vi "Search_Dust_Types.vi"() -> ()   [LabVIEW 2013]
doc: "Searches the dust_type table for a user-selected dust name. For use in the Dust Lab. All results can be ordered by id_dust_type, dust name, density, source mass, bottle mass, or dust mass."
uses:
  <userlib>/Accelerator/User Interface/Controls/Dust_list.ctl
  <vilib>/Utility/miscctls.llb/LVPointTypeDef.ctl
panel:
  out "Descending":string
  out "Ascending":string
  out "dust_weight text":string
  out "bottle_weight text":string
  out "source_weight text":string
  out "dust_density text":string
  out "dust_name text":string
  out "id_dust_type text":string
  in  "Exit":bool
  out "error out":errorcluster
  in  "error in (no error)":errorcluster
  in  "dust_weight":bool
  in  "bottle_weight":bool
  in  "source_weight":bool
  in  "dust_density":bool
  in  "dust_name":bool
  in  "id_dust_type":bool
  out "Array":T1[](array[typedef])
  # "Size"
  # "Comments"
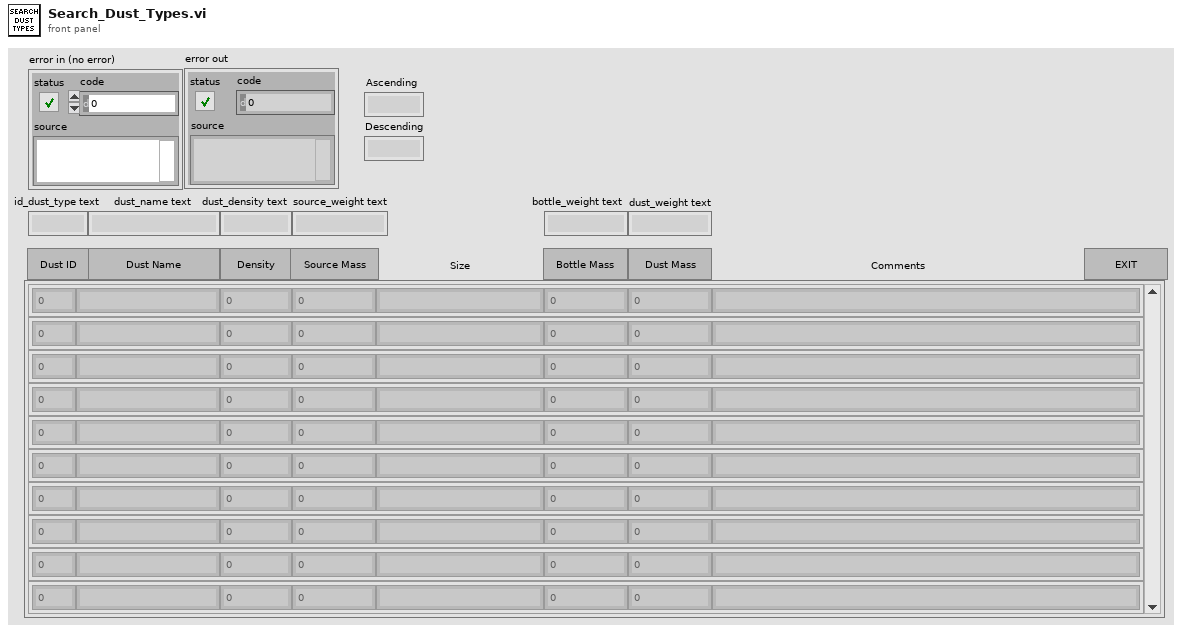
[diagram p1: front panel]
types:
  T1 = typedef "Dust_list.ctl" = cluster{"id_dust_type":i32, "dust_name":string, "dust_type":i32, "batch_no":i32, "dust_density":dbl, "source_weight":dbl, "size":string, "bottle_weight":dbl, "dust_mass":dbl, "comments":string}
  T2 = typedef "LVPointTypeDef.ctl" = cluster{"Horizontal":i16, "Vertical":i16}
  T3 = enum16{"dust_name", "dust_density", "source_weight", "bottle_weight", "dust_weight"}
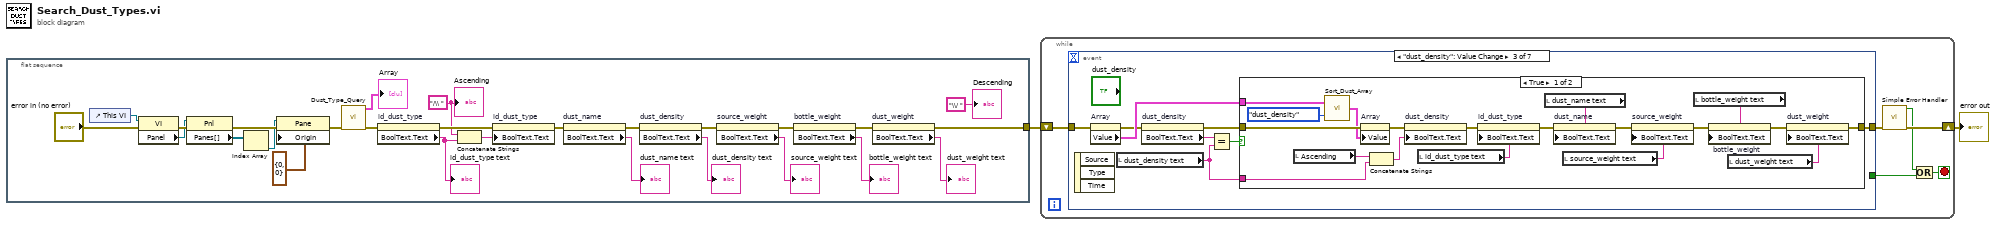
[diagram p0: block diagram]
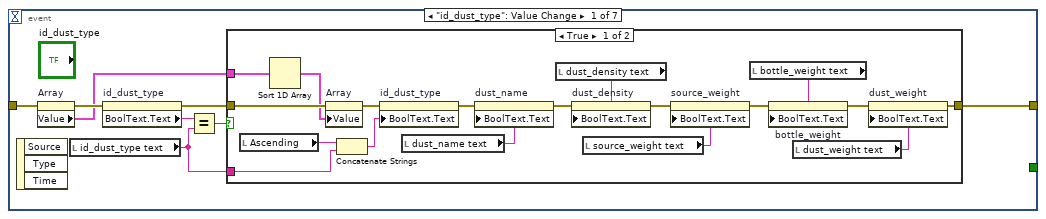
[diagram p2: hidden frame]
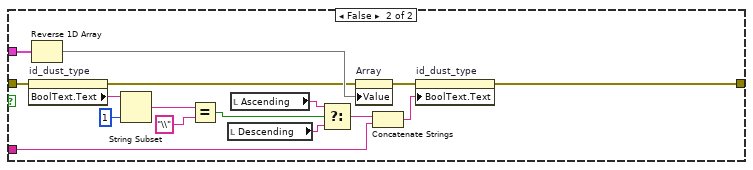
[diagram p3: hidden frame]
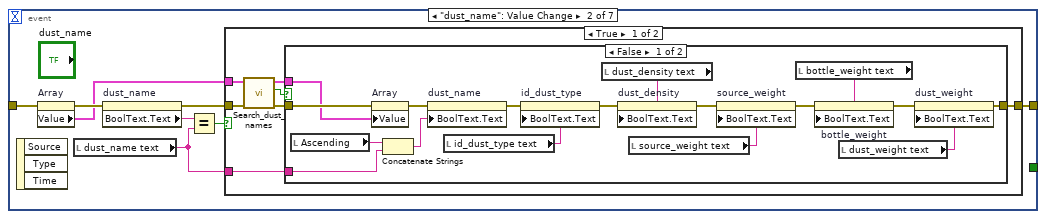
[diagram p4: hidden frame]
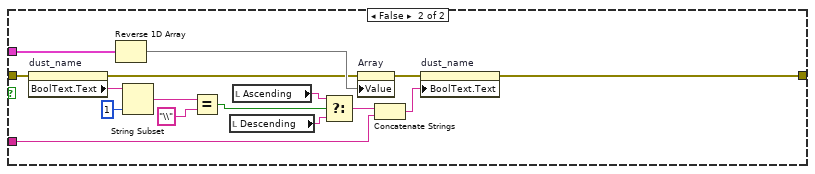
[diagram p6: hidden frame]
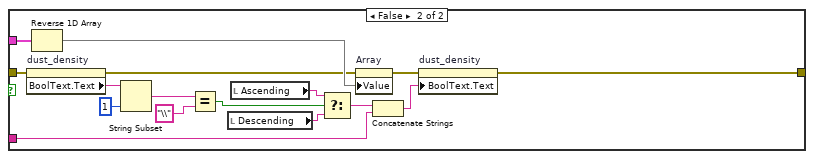
[diagram p7: hidden frame]
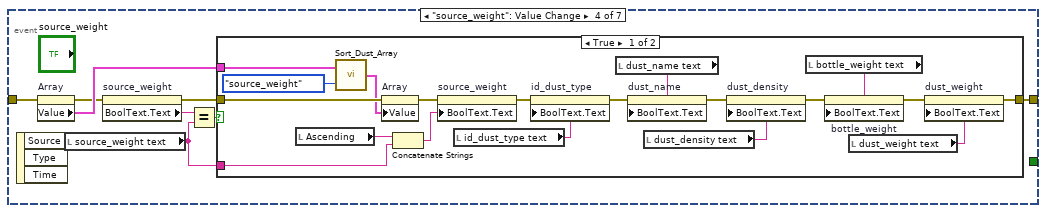
[diagram p8: hidden frame]
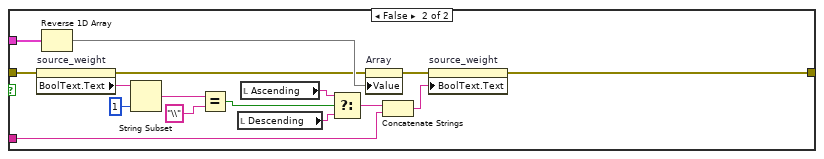
[diagram p9: hidden frame]
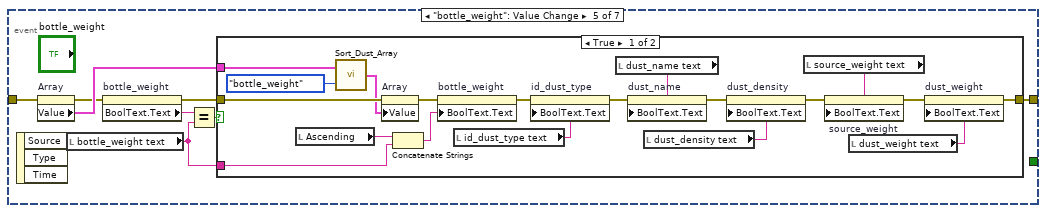
[diagram p10: hidden frame]
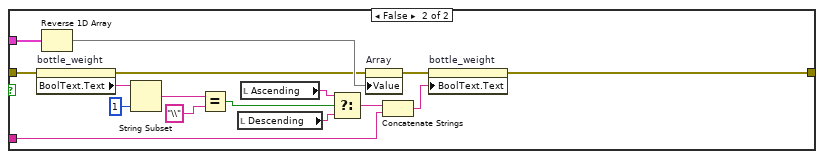
[diagram p11: hidden frame]
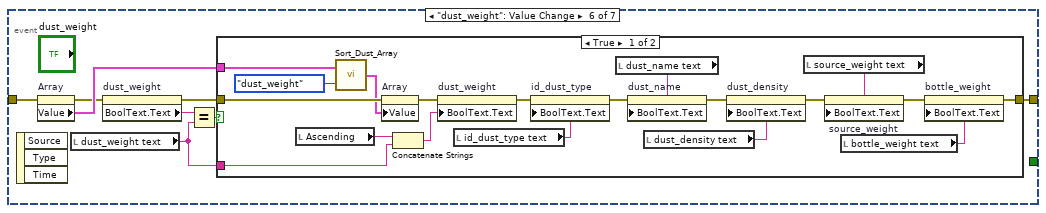
[diagram p12: hidden frame]
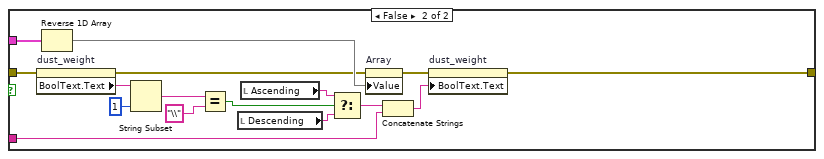
[diagram p13: hidden frame]
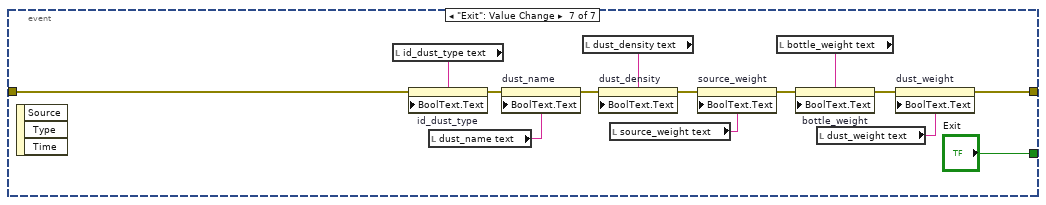
[diagram p14: hidden frame]
diagram:
  n1 = flat-sequence {
    tunnel: [w20] -> w1
    frame #0 {
      w3 = "/\\ " ("Ascending")
      n2 = control-ref of="This VI"() -> (w15:refnum<vi>)
      n3 = property class="VI"(reference=w15, error in="error in (no error)") -> (error out=w14:errorcluster, "Panel"=w13:refnum<vi>)  [unwired: 1 out]
      n4 = property class="Pnl"(reference=w13, error in=w14) -> (error out=w12:errorcluster, "Panes[]"=w11:refnum<vi>[])  [unwired: 1 out]
      n5 = Index Array(array=w11) -> (element=w10:refnum<vi>)  [unwired: 1 in]
      n6 = property class="Pane"(reference=w10, error in=w12, "Origin"=T2 {"Horizontal"=0, "Vertical"=0}) -> (error out=w8:errorcluster)  [unwired: 1 out]
      n7 = call <userlib>:"Dust_Type_Query.vi"("error in (no error)"=w8) -> ("error out"=w18:errorcluster, "Dust Type Array"=→"Array":T1[])  [unwired: 9 in]
      n8 = property on="id_dust_type" class="Bool"(error in=w18) -> (error out=w6:errorcluster, "BoolText.Text"=w4:string)  [unwired: 1 in, 1 out]
      "id_dust_type text" <- w4
      n9 = Concatenate Strings(w3, w4) -> (w5:string)
      n10 = property on="id_dust_type" class="Bool"(error in=w6, "BoolText.Text"=w5) -> (error out=w7:errorcluster)  [unwired: 1 in, 1 out]
      n11 = property on="dust_name" class="Bool"(error in=w7) -> (error out=w29:errorcluster, "BoolText.Text"=→"dust_name text":string)  [unwired: 1 in, 1 out]
      n12 = property on="dust_density" class="Bool"(error in=w29) -> (error out=w26:errorcluster, "BoolText.Text"=→"dust_density text":string)  [unwired: 1 in, 1 out]
      n13 = property on="source_weight" class="Bool"(error in=w26) -> (error out=w24:errorcluster, "BoolText.Text"=→"source_weight text":string)  [unwired: 1 in, 1 out]
      n14 = property on="bottle_weight" class="Bool"(error in=w24) -> (error out=w22:errorcluster, "BoolText.Text"=→"bottle_weight text":string)  [unwired: 1 in, 1 out]
      n15 = property on="dust_weight" class="Bool"(error in=w22) -> (error out=w20:errorcluster, "BoolText.Text"=→"dust_weight text":string)  [unwired: 1 in, 1 out]
      "Ascending" <- w3
      "Descending" <- "\\/ " ("Descending")
    }
  }
  n16 = while {
    shift-right: [w32] -> w2
    shift-left: w1 -> [w35]
    stop <- w31 stop-if-true
    n17 = event shown="[2] \"dust_density\": Value Change" {
      selector: _ -> [_ _ _ _ _ _ _]
      dyn-events: _ -> [_ _ _ _ _ _ _]
      timeout: _ -> [_ _ _ _ _ _ _]
      tunnel: w35 -> [w43 w85 w134 w177 w220 w263 w306]
      tunnel: [w42 w84 w133 w176 w219 w262 w305] -> w34
      tunnel: [_ _ _ _ _ _ "Exit"] -> w33
      event "id_dust_type": Value Change {
        n18 = event-data() -> ()  [unwired: 1 in, 3 out]
        n19 = property on="Array" class="Arr (strict)"(error in=w43) -> (error out=w37:errorcluster, "Value"=w36:T1[])  [unwired: 1 in, 1 out]
        n20 = local read "id_dust_type text"() -> (w40:string)
        n21 = property on="id_dust_type" class="Bool"(error in=w37) -> (error out=w38:errorcluster, "BoolText.Text"=w41:string)  [unwired: 1 in, 1 out]
        n22 = Equal?(x=w41, y=w40) -> (x = y?=w39:bool)
        n23 = case shown="True" w39 {
          tunnel: [w48 w76] -> w42
          tunnel: w40 -> [w59 w75]
          tunnel: w38 -> [w47 w64]
          tunnel: w36 -> [w45 w74]
          frame True {
            n24 = local read "Ascending"() -> (w60:string)
            n25 = Sort 1D Array(array=w45) -> (sorted array=w44:T1[])
            n26 = property on="Array" class="Arr (strict)"(error in=w47, "Value"=w44) -> (error out=w46:errorcluster)  [unwired: 1 in, 1 out]
            n27 = Concatenate Strings(w60, w59) -> (w61:string)
            n28 = property on="id_dust_type" class="Bool"(error in=w46, "BoolText.Text"=w61) -> (error out=w49:errorcluster)  [unwired: 1 in, 1 out]
            n29 = local read "dust_name text"() -> (w53:string)
            n30 = property on="dust_name" class="Bool"(error in=w49, "BoolText.Text"=w53) -> (error out=w54:errorcluster)  [unwired: 1 in, 1 out]
            n31 = local read "dust_density text"() -> (w52:string)
            n32 = property on="dust_density" class="Bool"(error in=w54, "BoolText.Text"=w52) -> (error out=w55:errorcluster)  [unwired: 1 in, 1 out]
            n33 = local read "source_weight text"() -> (w51:string)
            n34 = property on="source_weight" class="Bool"(error in=w55, "BoolText.Text"=w51) -> (error out=w56:errorcluster)  [unwired: 1 in, 1 out]
            n35 = local read "bottle_weight text"() -> (w50:string)
            n36 = property on="bottle_weight" class="Bool"(error in=w56, "BoolText.Text"=w50) -> (error out=w57:errorcluster)  [unwired: 1 in, 1 out]
            n37 = local read "dust_weight text"() -> (w58:string)
            n38 = property on="dust_weight" class="Bool"(error in=w57, "BoolText.Text"=w58) -> (error out=w48:errorcluster)  [unwired: 1 in, 1 out]
          }
          frame False {
            n39 = property on="id_dust_type" class="Bool"(error in=w64) -> (error out=w63:errorcluster, "BoolText.Text"=w70:string)  [unwired: 1 in, 1 out]
            n40 = Reverse 1D Array(array=w74) -> (reversed array=w73:T1[])
            n41 = String Subset(string=w70, length (rest)=1 ("length (rest)")) -> (substring=w67:string)  [unwired: 1 in]
            n42 = Equal?(x=w67, y="\\") -> (x = y?=w65:bool)
            n43 = local read "Descending"() -> (w72:string)
            n44 = local read "Ascending"() -> (w68:string)
            n45 = Select(t=w68, s=w65, f=w72) -> (s? t:f=w71:string)
            n46 = property on="Array" class="Arr (strict)"(error in=w63, "Value"=w73) -> (error out=w62:errorcluster)  [unwired: 1 in, 1 out]
            n47 = Concatenate Strings(w71, w75) -> (w77:string)
            n48 = property on="id_dust_type" class="Bool"(error in=w62, "BoolText.Text"=w77) -> (error out=w76:errorcluster)  [unwired: 1 in, 1 out]
          }
        }
      }
      event "dust_name": Value Change {
        n49 = event-data() -> ()  [unwired: 1 in, 3 out]
        n50 = property on="Array" class="Arr (strict)"(error in=w85) -> (error out=w81:errorcluster, "Value"=w79:T1[])  [unwired: 1 in, 1 out]
        n51 = local read "dust_name text"() -> (w83:string)
        n52 = property on="dust_name" class="Bool"(error in=w81) -> (error out=w78:errorcluster, "BoolText.Text"=w80:string)  [unwired: 1 in, 1 out]
        n53 = Equal?(x=w80, y=w83) -> (x = y?=w82:bool)
        n54 = case shown="True" w82 {
          tunnel: [w91 w112] -> w84
          tunnel: w83 -> [w92 w126]
          tunnel: w78 -> [w90 w116]
          tunnel: w79 -> [w88 w125]
          frame True {
            n55 = call <userlib>:"Search_dust_names.vi"("error in (no error)"=w90, "Dust array in"=w88) -> ("error out"=w89:errorcluster, "Cancelled?"=w86:bool, "Dust array out"=w87:T1[])  [unwired: 7 in]
            n56 = case shown="False" w86 {
              tunnel: w92 -> [w108 _]
              tunnel: [w98 w110] -> w91
              tunnel: w89 -> [w94 w110]
              tunnel: w87 -> [w93 _]
              frame False {
                n57 = local read "Ascending"() -> (w109:string)
                n58 = property on="Array" class="Arr (strict)"(error in=w94, "Value"=w93) -> (error out=w96:errorcluster)  [unwired: 1 in, 1 out]
                n59 = Concatenate Strings(w109, w108) -> (w95:string)
                n60 = property on="dust_name" class="Bool"(error in=w96, "BoolText.Text"=w95) -> (error out=w97:errorcluster)  [unwired: 1 in, 1 out]
                n61 = local read "id_dust_type text"() -> (w102:string)
                n62 = property on="id_dust_type" class="Bool"(error in=w97, "BoolText.Text"=w102) -> (error out=w103:errorcluster)  [unwired: 1 in, 1 out]
                n63 = local read "dust_density text"() -> (w101:string)
                n64 = property on="dust_density" class="Bool"(error in=w103, "BoolText.Text"=w101) -> (error out=w104:errorcluster)  [unwired: 1 in, 1 out]
                n65 = local read "source_weight text"() -> (w100:string)
                n66 = property on="source_weight" class="Bool"(error in=w104, "BoolText.Text"=w100) -> (error out=w105:errorcluster)  [unwired: 1 in, 1 out]
                n67 = local read "bottle_weight text"() -> (w99:string)
                n68 = property on="bottle_weight" class="Bool"(error in=w105, "BoolText.Text"=w99) -> (error out=w106:errorcluster)  [unwired: 1 in, 1 out]
                n69 = local read "dust_weight text"() -> (w107:string)
                n70 = property on="dust_weight" class="Bool"(error in=w106, "BoolText.Text"=w107) -> (error out=w98:errorcluster)  [unwired: 1 in, 1 out]
              }
              frame True {
              }
            }
          }
          frame False {
            n71 = property on="dust_name" class="Bool"(error in=w116) -> (error out=w115:errorcluster, "BoolText.Text"=w114:string)  [unwired: 1 in, 1 out]
            n72 = Reverse 1D Array(array=w125) -> (reversed array=w124:T1[])
            n73 = String Subset(string=w114, length (rest)=1 ("length (rest)")) -> (substring=w119:string)  [unwired: 1 in]
            n74 = Equal?(x=w119, y="\\") -> (x = y?=w117:bool)
            n75 = local read "Descending"() -> (w123:string)
            n76 = local read "Ascending"() -> (w120:string)
            n77 = Select(t=w120, s=w117, f=w123) -> (s? t:f=w122:string)
            n78 = property on="Array" class="Arr (strict)"(error in=w115, "Value"=w124) -> (error out=w113:errorcluster)  [unwired: 1 in, 1 out]
            n79 = Concatenate Strings(w122, w126) -> (w111:string)
            n80 = property on="dust_name" class="Bool"(error in=w113, "BoolText.Text"=w111) -> (error out=w112:errorcluster)  [unwired: 1 in, 1 out]
          }
        }
      }
      event "dust_density": Value Change {
        n81 = event-data() -> ()  [unwired: 1 in, 3 out]
        n82 = property on="Array" class="Arr (strict)"(error in=w134) -> (error out=w129:errorcluster, "Value"=w130:T1[])  [unwired: 1 in, 1 out]
        n83 = local read "dust_density text"() -> (w132:string)
        n84 = property on="dust_density" class="Bool"(error in=w129) -> (error out=w127:errorcluster, "BoolText.Text"=w128:string)  [unwired: 1 in, 1 out]
        n85 = Equal?(x=w128, y=w132) -> (x = y?=w131:bool)
        n86 = case shown="True" w131 {
          tunnel: [w142 w155] -> w133
          tunnel: w132 -> [w152 w169]
          tunnel: w127 -> [w141 w159]
          tunnel: w130 -> [w140 w168]
          frame True {
            n87 = local read "Ascending"() -> (w153:string)
            n88 = call <userlib>:"Sort_Dust_Array.vi"("Order by..."=T3."dust_density", "Array In"=w140) -> ("Array out"=w139:T1[])
            n89 = property on="Array" class="Arr (strict)"(error in=w141, "Value"=w139) -> (error out=w137:errorcluster)  [unwired: 1 in, 1 out]
            n90 = Concatenate Strings(w153, w152) -> (w136:string)
            n91 = property on="dust_density" class="Bool"(error in=w137, "BoolText.Text"=w136) -> (error out=w138:errorcluster)  [unwired: 1 in, 1 out]
            n92 = local read "id_dust_type text"() -> (w146:string)
            n93 = property on="id_dust_type" class="Bool"(error in=w138, "BoolText.Text"=w146) -> (error out=w147:errorcluster)  [unwired: 1 in, 1 out]
            n94 = local read "dust_name text"() -> (w145:string)
            n95 = property on="dust_name" class="Bool"(error in=w147, "BoolText.Text"=w145) -> (error out=w148:errorcluster)  [unwired: 1 in, 1 out]
            n96 = local read "source_weight text"() -> (w144:string)
            n97 = property on="source_weight" class="Bool"(error in=w148, "BoolText.Text"=w144) -> (error out=w149:errorcluster)  [unwired: 1 in, 1 out]
            n98 = local read "bottle_weight text"() -> (w143:string)
            n99 = property on="bottle_weight" class="Bool"(error in=w149, "BoolText.Text"=w143) -> (error out=w150:errorcluster)  [unwired: 1 in, 1 out]
            n100 = local read "dust_weight text"() -> (w151:string)
            n101 = property on="dust_weight" class="Bool"(error in=w150, "BoolText.Text"=w151) -> (error out=w142:errorcluster)  [unwired: 1 in, 1 out]
          }
          frame False {
            n102 = property on="dust_density" class="Bool"(error in=w159) -> (error out=w158:errorcluster, "BoolText.Text"=w157:string)  [unwired: 1 in, 1 out]
            n103 = Reverse 1D Array(array=w168) -> (reversed array=w167:T1[])
            n104 = String Subset(string=w157, length (rest)=1 ("length (rest)")) -> (substring=w162:string)  [unwired: 1 in]
            n105 = Equal?(x=w162, y="\\") -> (x = y?=w160:bool)
            n106 = local read "Descending"() -> (w166:string)
            n107 = local read "Ascending"() -> (w163:string)
            n108 = Select(t=w163, s=w160, f=w166) -> (s? t:f=w165:string)
            n109 = property on="Array" class="Arr (strict)"(error in=w158, "Value"=w167) -> (error out=w156:errorcluster)  [unwired: 1 in, 1 out]
            n110 = Concatenate Strings(w165, w169) -> (w154:string)
            n111 = property on="dust_density" class="Bool"(error in=w156, "BoolText.Text"=w154) -> (error out=w155:errorcluster)  [unwired: 1 in, 1 out]
          }
        }
      }
      event "source_weight": Value Change {
        n112 = event-data() -> ()  [unwired: 1 in, 3 out]
        n113 = property on="Array" class="Arr (strict)"(error in=w177) -> (error out=w172:errorcluster, "Value"=w173:T1[])  [unwired: 1 in, 1 out]
        n114 = local read "source_weight text"() -> (w175:string)
        n115 = property on="source_weight" class="Bool"(error in=w172) -> (error out=w170:errorcluster, "BoolText.Text"=w171:string)  [unwired: 1 in, 1 out]
        n116 = Equal?(x=w171, y=w175) -> (x = y?=w174:bool)
        n117 = case shown="True" w174 {
          tunnel: [w185 w198] -> w176
          tunnel: w175 -> [w195 w212]
          tunnel: w170 -> [w184 w202]
          tunnel: w173 -> [w183 w211]
          frame True {
            n118 = local read "Ascending"() -> (w196:string)
            n119 = call <userlib>:"Sort_Dust_Array.vi"("Order by..."=T3."source_weight", "Array In"=w183) -> ("Array out"=w182:T1[])
            n120 = property on="Array" class="Arr (strict)"(error in=w184, "Value"=w182) -> (error out=w180:errorcluster)  [unwired: 1 in, 1 out]
            n121 = Concatenate Strings(w196, w195) -> (w179:string)
            n122 = property on="source_weight" class="Bool"(error in=w180, "BoolText.Text"=w179) -> (error out=w181:errorcluster)  [unwired: 1 in, 1 out]
            n123 = local read "id_dust_type text"() -> (w189:string)
            n124 = property on="id_dust_type" class="Bool"(error in=w181, "BoolText.Text"=w189) -> (error out=w190:errorcluster)  [unwired: 1 in, 1 out]
            n125 = local read "dust_name text"() -> (w188:string)
            n126 = property on="dust_name" class="Bool"(error in=w190, "BoolText.Text"=w188) -> (error out=w191:errorcluster)  [unwired: 1 in, 1 out]
            n127 = local read "dust_density text"() -> (w187:string)
            n128 = property on="dust_density" class="Bool"(error in=w191, "BoolText.Text"=w187) -> (error out=w192:errorcluster)  [unwired: 1 in, 1 out]
            n129 = local read "bottle_weight text"() -> (w186:string)
            n130 = property on="bottle_weight" class="Bool"(error in=w192, "BoolText.Text"=w186) -> (error out=w193:errorcluster)  [unwired: 1 in, 1 out]
            n131 = local read "dust_weight text"() -> (w194:string)
            n132 = property on="dust_weight" class="Bool"(error in=w193, "BoolText.Text"=w194) -> (error out=w185:errorcluster)  [unwired: 1 in, 1 out]
          }
          frame False {
            n133 = property on="source_weight" class="Bool"(error in=w202) -> (error out=w201:errorcluster, "BoolText.Text"=w200:string)  [unwired: 1 in, 1 out]
            n134 = Reverse 1D Array(array=w211) -> (reversed array=w210:T1[])
            n135 = String Subset(string=w200, length (rest)=1 ("length (rest)")) -> (substring=w205:string)  [unwired: 1 in]
            n136 = Equal?(x=w205, y="\\") -> (x = y?=w203:bool)
            n137 = local read "Descending"() -> (w209:string)
            n138 = local read "Ascending"() -> (w206:string)
            n139 = Select(t=w206, s=w203, f=w209) -> (s? t:f=w208:string)
            n140 = property on="Array" class="Arr (strict)"(error in=w201, "Value"=w210) -> (error out=w199:errorcluster)  [unwired: 1 in, 1 out]
            n141 = Concatenate Strings(w208, w212) -> (w197:string)
            n142 = property on="source_weight" class="Bool"(error in=w199, "BoolText.Text"=w197) -> (error out=w198:errorcluster)  [unwired: 1 in, 1 out]
          }
        }
      }
      event "bottle_weight": Value Change {
        n143 = event-data() -> ()  [unwired: 1 in, 3 out]
        n144 = property on="Array" class="Arr (strict)"(error in=w220) -> (error out=w215:errorcluster, "Value"=w216:T1[])  [unwired: 1 in, 1 out]
        n145 = local read "bottle_weight text"() -> (w218:string)
        n146 = property on="bottle_weight" class="Bool"(error in=w215) -> (error out=w213:errorcluster, "BoolText.Text"=w214:string)  [unwired: 1 in, 1 out]
        n147 = Equal?(x=w214, y=w218) -> (x = y?=w217:bool)
        n148 = case shown="True" w217 {
          tunnel: [w228 w241] -> w219
          tunnel: w218 -> [w238 w255]
          tunnel: w213 -> [w227 w245]
          tunnel: w216 -> [w226 w254]
          frame True {
            n149 = local read "Ascending"() -> (w239:string)
            n150 = call <userlib>:"Sort_Dust_Array.vi"("Order by..."=T3."bottle_weight", "Array In"=w226) -> ("Array out"=w225:T1[])
            n151 = property on="Array" class="Arr (strict)"(error in=w227, "Value"=w225) -> (error out=w223:errorcluster)  [unwired: 1 in, 1 out]
            n152 = Concatenate Strings(w239, w238) -> (w222:string)
            n153 = property on="bottle_weight" class="Bool"(error in=w223, "BoolText.Text"=w222) -> (error out=w224:errorcluster)  [unwired: 1 in, 1 out]
            n154 = local read "id_dust_type text"() -> (w232:string)
            n155 = property on="id_dust_type" class="Bool"(error in=w224, "BoolText.Text"=w232) -> (error out=w233:errorcluster)  [unwired: 1 in, 1 out]
            n156 = local read "dust_name text"() -> (w231:string)
            n157 = property on="dust_name" class="Bool"(error in=w233, "BoolText.Text"=w231) -> (error out=w234:errorcluster)  [unwired: 1 in, 1 out]
            n158 = local read "dust_density text"() -> (w230:string)
            n159 = property on="dust_density" class="Bool"(error in=w234, "BoolText.Text"=w230) -> (error out=w235:errorcluster)  [unwired: 1 in, 1 out]
            n160 = local read "source_weight text"() -> (w229:string)
            n161 = property on="source_weight" class="Bool"(error in=w235, "BoolText.Text"=w229) -> (error out=w236:errorcluster)  [unwired: 1 in, 1 out]
            n162 = local read "dust_weight text"() -> (w237:string)
            n163 = property on="dust_weight" class="Bool"(error in=w236, "BoolText.Text"=w237) -> (error out=w228:errorcluster)  [unwired: 1 in, 1 out]
          }
          frame False {
            n164 = property on="bottle_weight" class="Bool"(error in=w245) -> (error out=w244:errorcluster, "BoolText.Text"=w243:string)  [unwired: 1 in, 1 out]
            n165 = Reverse 1D Array(array=w254) -> (reversed array=w253:T1[])
            n166 = String Subset(string=w243, length (rest)=1 ("length (rest)")) -> (substring=w248:string)  [unwired: 1 in]
            n167 = Equal?(x=w248, y="\\") -> (x = y?=w246:bool)
            n168 = local read "Descending"() -> (w252:string)
            n169 = local read "Ascending"() -> (w249:string)
            n170 = Select(t=w249, s=w246, f=w252) -> (s? t:f=w251:string)
            n171 = property on="Array" class="Arr (strict)"(error in=w244, "Value"=w253) -> (error out=w242:errorcluster)  [unwired: 1 in, 1 out]
            n172 = Concatenate Strings(w251, w255) -> (w240:string)
            n173 = property on="bottle_weight" class="Bool"(error in=w242, "BoolText.Text"=w240) -> (error out=w241:errorcluster)  [unwired: 1 in, 1 out]
          }
        }
      }
      event "dust_weight": Value Change {
        n174 = event-data() -> ()  [unwired: 1 in, 3 out]
        n175 = property on="Array" class="Arr (strict)"(error in=w263) -> (error out=w258:errorcluster, "Value"=w259:T1[])  [unwired: 1 in, 1 out]
        n176 = local read "dust_weight text"() -> (w261:string)
        n177 = property on="dust_weight" class="Bool"(error in=w258) -> (error out=w256:errorcluster, "BoolText.Text"=w257:string)  [unwired: 1 in, 1 out]
        n178 = Equal?(x=w257, y=w261) -> (x = y?=w260:bool)
        n179 = case shown="True" w260 {
          tunnel: [w271 w284] -> w262
          tunnel: w261 -> [w281 w298]
          tunnel: w256 -> [w270 w288]
          tunnel: w259 -> [w269 w297]
          frame True {
            n180 = local read "Ascending"() -> (w282:string)
            n181 = call <userlib>:"Sort_Dust_Array.vi"("Order by..."=T3."dust_weight", "Array In"=w269) -> ("Array out"=w268:T1[])
            n182 = property on="Array" class="Arr (strict)"(error in=w270, "Value"=w268) -> (error out=w266:errorcluster)  [unwired: 1 in, 1 out]
            n183 = Concatenate Strings(w282, w281) -> (w265:string)
            n184 = property on="dust_weight" class="Bool"(error in=w266, "BoolText.Text"=w265) -> (error out=w267:errorcluster)  [unwired: 1 in, 1 out]
            n185 = local read "id_dust_type text"() -> (w275:string)
            n186 = property on="id_dust_type" class="Bool"(error in=w267, "BoolText.Text"=w275) -> (error out=w276:errorcluster)  [unwired: 1 in, 1 out]
            n187 = local read "dust_name text"() -> (w274:string)
            n188 = property on="dust_name" class="Bool"(error in=w276, "BoolText.Text"=w274) -> (error out=w277:errorcluster)  [unwired: 1 in, 1 out]
            n189 = local read "dust_density text"() -> (w273:string)
            n190 = property on="dust_density" class="Bool"(error in=w277, "BoolText.Text"=w273) -> (error out=w278:errorcluster)  [unwired: 1 in, 1 out]
            n191 = local read "source_weight text"() -> (w272:string)
            n192 = property on="source_weight" class="Bool"(error in=w278, "BoolText.Text"=w272) -> (error out=w279:errorcluster)  [unwired: 1 in, 1 out]
            n193 = local read "bottle_weight text"() -> (w280:string)
            n194 = property on="bottle_weight" class="Bool"(error in=w279, "BoolText.Text"=w280) -> (error out=w271:errorcluster)  [unwired: 1 in, 1 out]
          }
          frame False {
            n195 = property on="dust_weight" class="Bool"(error in=w288) -> (error out=w287:errorcluster, "BoolText.Text"=w286:string)  [unwired: 1 in, 1 out]
            n196 = Reverse 1D Array(array=w297) -> (reversed array=w296:T1[])
            n197 = String Subset(string=w286, length (rest)=1 ("length (rest)")) -> (substring=w291:string)  [unwired: 1 in]
            n198 = Equal?(x=w291, y="\\") -> (x = y?=w289:bool)
            n199 = local read "Descending"() -> (w295:string)
            n200 = local read "Ascending"() -> (w292:string)
            n201 = Select(t=w292, s=w289, f=w295) -> (s? t:f=w294:string)
            n202 = property on="Array" class="Arr (strict)"(error in=w287, "Value"=w296) -> (error out=w285:errorcluster)  [unwired: 1 in, 1 out]
            n203 = Concatenate Strings(w294, w298) -> (w283:string)
            n204 = property on="dust_weight" class="Bool"(error in=w285, "BoolText.Text"=w283) -> (error out=w284:errorcluster)  [unwired: 1 in, 1 out]
          }
        }
      }
      event "Exit": Value Change {
        n205 = event-data() -> ()  [unwired: 1 in, 3 out]
        n206 = local read "id_dust_type text"() -> (w304:string)
        n207 = property on="id_dust_type" class="Bool"(error in=w306, "BoolText.Text"=w304) -> (error out=w307:errorcluster)  [unwired: 1 in, 1 out]
        n208 = local read "dust_name text"() -> (w303:string)
        n209 = property on="dust_name" class="Bool"(error in=w307, "BoolText.Text"=w303) -> (error out=w308:errorcluster)  [unwired: 1 in, 1 out]
        n210 = local read "dust_density text"() -> (w302:string)
        n211 = property on="dust_density" class="Bool"(error in=w308, "BoolText.Text"=w302) -> (error out=w309:errorcluster)  [unwired: 1 in, 1 out]
        n212 = local read "source_weight text"() -> (w301:string)
        n213 = property on="source_weight" class="Bool"(error in=w309, "BoolText.Text"=w301) -> (error out=w310:errorcluster)  [unwired: 1 in, 1 out]
        n214 = local read "bottle_weight text"() -> (w300:string)
        n215 = property on="bottle_weight" class="Bool"(error in=w310, "BoolText.Text"=w300) -> (error out=w311:errorcluster)  [unwired: 1 in, 1 out]
        n216 = local read "dust_weight text"() -> (w299:string)
        n217 = property on="dust_weight" class="Bool"(error in=w311, "BoolText.Text"=w299) -> (error out=w305:errorcluster)  [unwired: 1 in, 1 out]
      }
    }
    n218 = call <vilib>:"Simple Error Handler.vi"("error in (no error)"=w34) -> ("error?"=w30:bool, "error out"=w32:errorcluster)  [unwired: 4 in, 3 out]
    n219 = Or(x=w30, y=w33) -> (x .or. y?=w31:bool)
  }
  "error out" <- w2
